vi "Database.vi"(7 "Database Action":T2, 11 "User":T1) -> (2 "Database":T1[](array[typedef]))   [LabVIEW 2020]
uses:
  #typedef_DatabaseAction.ctl
  #typedef_Student.ctl
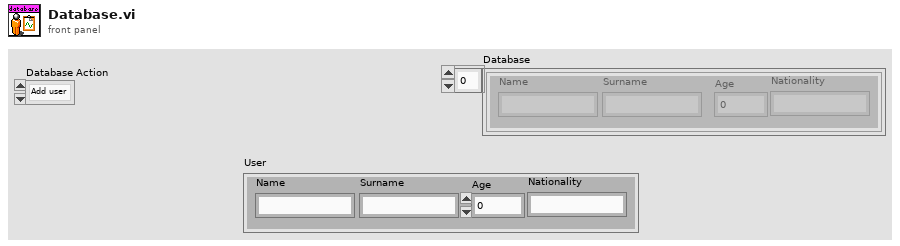
[diagram p1: front panel]
types:
  T1 = typedef "#typedef_Student.ctl" = cluster{"Name":string, "Surname":string, "Age":dbl, "Nationality":string}
  T2 = typedef "#typedef_DatabaseAction.ctl" = enum16{"Add user", "Get database", "Clear database"}
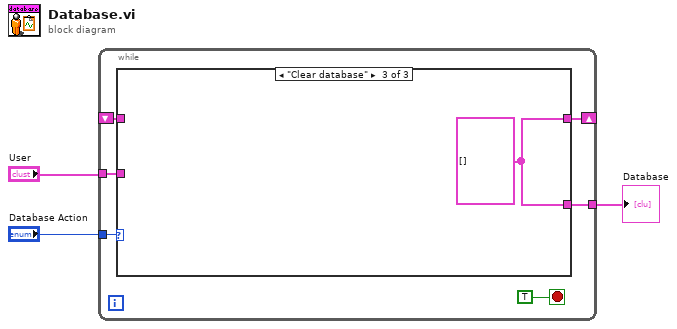
[diagram p0: block diagram]
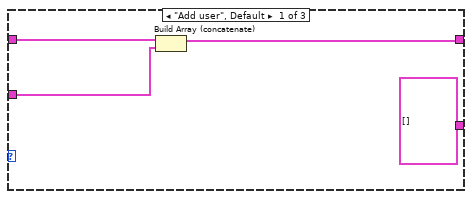
[diagram p2: hidden frame]
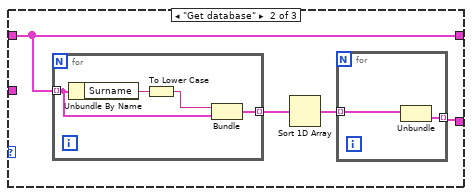
[diagram p3: hidden frame]
diagram:
  n1 = while {
    tunnel: "Database Action" -> [w8]
    shift-right: [w6] -> _
    shift-left: _ -> [w7]
    tunnel: "User" -> [w5]
    tunnel: [w4] -> w1
    stop <- TRUE stop-if-true
    n2 = case shown="\"Clear database\"" w8 {
      tunnel: w7 -> [w13 w14 _]
      tunnel: [w12 w14 w24] -> w6
      tunnel: w5 -> [w11 _ _]
      tunnel: [T1[] [] w15 w24] -> w4
      frame "Add user", Default {
        n3 = Build Array (concatenate)(w13, w11) -> (w12:T1[])
      }
      frame "Get database" {
        n4 = for {
          tunnel: w14 -> [w23] mode=indexing
          tunnel: [w22] -> w17 mode=indexing
          n5 = Unbundle By Name(w23) -> ("Surname"=w21:string)
          n6 = To Lower Case(string=w21) -> (all lower case string=w20:string)
          n7 = Bundle(w20, "Student"=w23) -> (w22:cluster{string, "Student":T1})  [unwired: 1 in]
        }
        n8 = Sort 1D Array(array=w17) -> (sorted array=w16:cluster{string, "Student":T1}[])
        n9 = for {
          tunnel: w16 -> [w19] mode=indexing
          tunnel: [w18] -> w15 mode=indexing
          n10 = Unbundle(w19) -> ("Student"=w18:T1)  [unwired: 1 out]
        }
      }
      frame "Clear database" {
        w24 = T1[] []
      }
    }
  }
  "Database" <- w1
